vi "RSZVB Write To Instrument.vi"(8 "error in (no error)":errorcluster {"code" format="%.0x"}, 10 "Write Buffer (*RST)":string="*RST", 11 "VISA session":refnum<visa-resource-name>) -> (0 "error out":errorcluster {"code" format="%.0x"}, 3 "dup VISA session":refnum<visa-resource-name>)   [LabVIEW 2011]
doc: "This VI writes commands and queries to the instrument to modify parameters and query device settings."
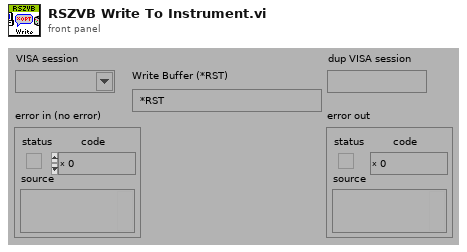
[diagram p1: front panel]
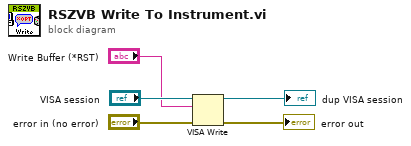
[diagram p0: block diagram]
diagram:
  n1 = VISA Write(VISA resource name="VISA session", write buffer="Write Buffer (*RST)", error in (no error)="error in (no error)") -> (VISA resource name out=→"dup VISA session":refnum<visa-resource-name>, error out=→"error out":errorcluster)  [unwired: 1 out]
